vi "Write CMD_IDENTIFICATION.vi"(8 "error in (no error)":errorcluster, 10 "CMD_IDENTIFICATION":u8, 11 "SMSD ADU in":refnum<class "SMSD ADU.lvclass">) -> (0 "error out":errorcluster, 3 "SMSD ADU out":refnum<class "SMSD ADU.lvclass">)   [LabVIEW 2021, in "SMSD ADU.lvclass"]
uses:
  SMSD ADU.lvclass
  SMSD ADU.lvclass/SMSD ADU.ctl
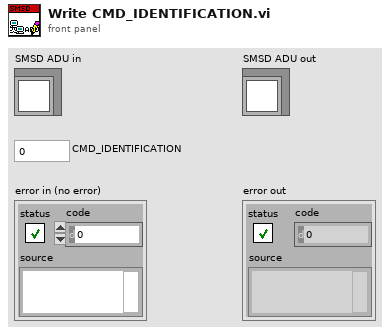
[diagram p1: front panel]
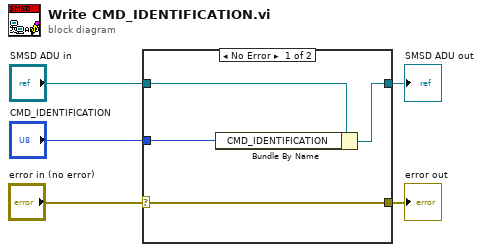
[diagram p0: block diagram]
diagram:
  n1 = case shown="No Error" "error in (no error)" {
    selector: "error in (no error)" -> [w6 w11]
    tunnel: "SMSD ADU in" -> [w9 w10]
    tunnel: [w8 w10] -> w4
    tunnel: "CMD_IDENTIFICATION" -> [w7 _]
    tunnel: [w6 w11] -> w1
    frame No Error {
      n2 = Bundle By Name(cluster=w9, "CMD_IDENTIFICATION"=w7) -> (w8:refnum<class "SMSD ADU.lvclass">)
    }
    frame Error {
    }
  }
  "SMSD ADU out" <- w4
  "error out" <- w1
